vi "steven 2.vi"() -> ()   [LabVIEW 2017]
panel:
  out "Meter":dbl(knob) scale=0.0..10.0
  out "Dial":cluster{dbl, dbl}(knob) scale=0.0..10.0
  in  "Knob":dbl(knob) scale=0.0..10.0
  out "Boolean":bool
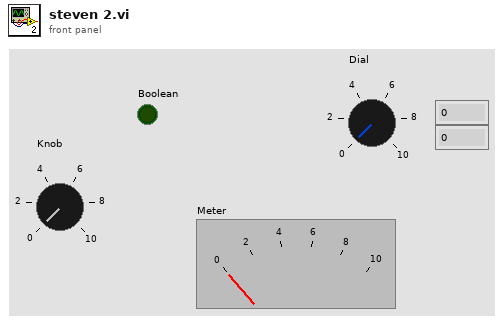
[diagram p1: front panel]
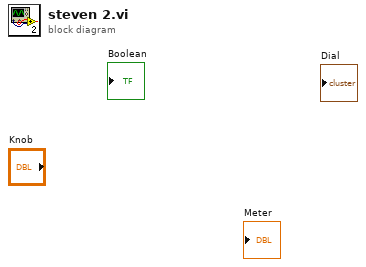
[diagram p0: block diagram]
diagram:
